vi "merFISH_uptade_scan_steps_indicators.vi"(2 "Total # steps":i32, 3 "scan step":i32) -> (0 "scan step":i32, 1 "slider":u8)   [LabVIEW 2015]
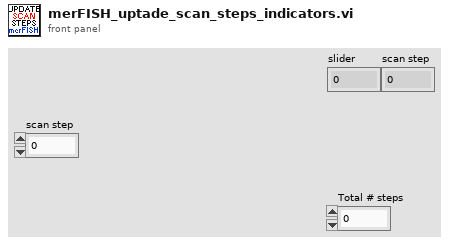
[diagram p1: front panel]
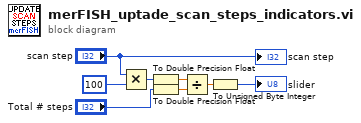
[diagram p0: block diagram]
diagram:
  n1 = Multiply(x="scan step", y=100) -> (x*y=w7:i32)
  n2 = To Double Precision Float(number=w7) -> (double precision float=w3:dbl)
  n3 = To Double Precision Float(number="Total # steps") -> (double precision float=w2:dbl)
  n4 = Divide(x=w3, y=w2) -> (x/y=w6:dbl)
  n5 = To Unsigned Byte Integer(number=w6) -> (unsigned 8bit integer=→"slider":u8)
  "scan step" <- "scan step"
